vi "Voltage to Total Test Energy.vi"(3 "PSU Voltage (kV)":dbl min=0.0 max=28000.0 format="%#_2p") -> (0 "Voltage Set":dbl, 1 "Total Energy of Test":dbl)   [LabVIEW 2015]
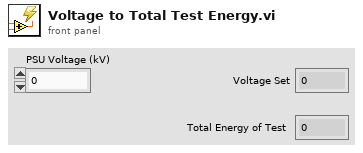
[diagram p1: front panel]
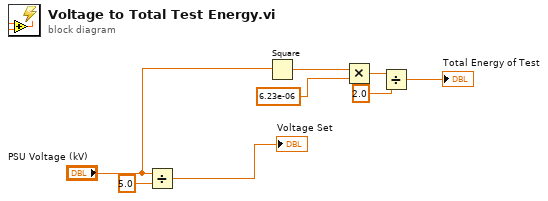
[diagram p0: block diagram]
diagram:
  n1 = Divide(x="PSU Voltage (kV)", y=5.0) -> (x/y=→"Voltage Set":dbl)
  n2 = Square(x="PSU Voltage (kV)") -> (x^2=w8:dbl)
  n3 = Multiply(x=w8, y=6.23e-06) -> (x*y=w3:dbl)
  n4 = Divide(x=w3, y=2.0) -> (x/y=→"Total Energy of Test":dbl)
